vi "Draw.vi"(8 "error in (no error)":errorcluster, 10 "2D Picture in":picture, 11 "Triangle in":refnum<class "Triangle.lvclass">) -> (0 "error out":errorcluster, 2 "2D Picture out":picture, 3 "Triangle out":refnum<class "Triangle.lvclass">)   [LabVIEW 2021, in "Picture2D.lvlib" / "Triangle.lvclass"]
uses:
  Triangle.lvclass
  Triangle.lvclass/Triangle.ctl
  Polygone/Polygone.lvclass
  Color/Color.lvclass
  Point/Point.lvclass
  Pen/Pen.lvclass
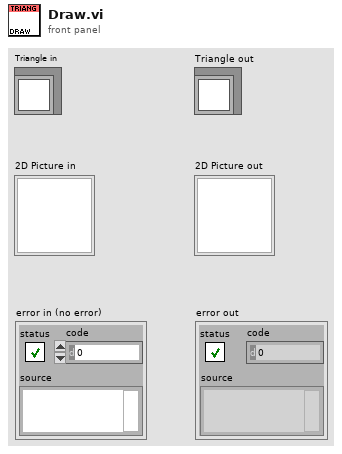
[diagram p1: front panel]
types:
  T1 = cluster{"Width":u16, "Style":enum32{"Solid", "Dash", "Dot", "DashDot", "DashDotDot"}}
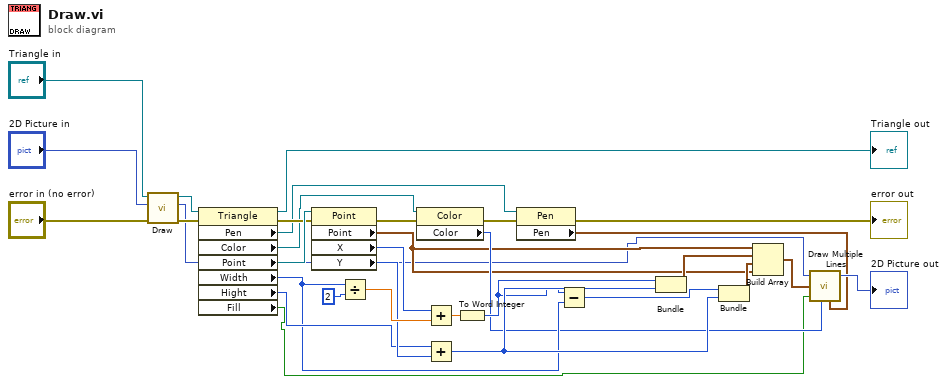
[diagram p0: block diagram]
diagram:
  n1 = call-parent "Draw.vi"("error in (no error)"="error in (no error)", "2D Picture in"="2D Picture in", "Shape in"="Triangle in") -> ("error out"=w18:errorcluster, "2D Picture out"=w3:picture, "Shape out"=w29:refnum<class "Triangle.lvclass">)  [unwired: 6 in]
  n2 = property class="Triangle"(reference=w29, error in=w18) -> (reference out=→"Triangle out":refnum<class "Triangle.lvclass">, error out=w21:errorcluster, "Pen"=w15:refnum<class "Pen.lvclass">, "Color"=w14:refnum<class "Color.lvclass">, "Point"=w28:refnum<class "Point.lvclass">, "Width"=w11:i16, "Hight"=w23:i16, "Fill"=w1:bool)
  n3 = property class="Point"(reference=w28, error in=w21) -> (error out=w20:errorcluster, "Point"=w5:cluster{"x":i16, "y":i16}, "X"=w26:i16, "Y"=w24:i16)  [unwired: 1 out]
  n4 = Divide(x=w11, y=i16 2) -> (x/y=w25:dbl)
  n5 = property class="Color"(reference=w14, error in=w20) -> (error out=w19:errorcluster, "Color"=w8:u32)  [unwired: 1 out]
  n6 = Add(x=w26, y=w25) -> (x+y=w22:dbl)
  n7 = Add(x=w23, y=w24) -> (x+y=w13:i16)
  n8 = To Word Integer(number=w22) -> (16bit integer=w12:i16)
  n9 = property class="Pen"(reference=w15, error in=w19) -> (error out=→"error out":errorcluster, "Pen"=w2:T1)  [unwired: 1 out]
  n10 = Subtract(x=w12, y=w11) -> (x-y=w10:i16)
  n11 = Bundle(w12, w13) -> (w7:cluster{i16, i16})  [unwired: 1 in]
  n12 = Bundle(w10, w13) -> (w6:cluster{i16, i16})  [unwired: 1 in]
  n13 = Build Array(w5, w7, w6, w5) -> (w4:cluster{"x":i16, "y":i16}[])
  n14 = call <vilib>:"Draw Multiple Lines.vi"("picture"=w3, "line endpoints"=w4, "fill?(F)"=w1, "color(black)"=w8, "pen"=w2) -> ("new picture"=→"2D Picture out":picture)  [unwired: 4 in]
